vi "Assert Greater_Variant.vi"(4 "Execution time (s)":dbl=-1.0, 6 "error code (1)":i32=1, 7 "Label":string, 8 "error in":errorcluster, 10 "Y":variant, 11 "X":variant) -> (0 "error out":errorcluster, 2 "Properties":refnum<class "Properties.Assert.lvclass">)   [LabVIEW 2021, in "Banana.Caraya.lvlib" / "Platano.CarayaTestSuite.lvclass"]
uses:
  Banana.Caraya/Platano.CarayaTestSuite/Platano.CarayaTestSuite.lvclass
  Banana.Caraya/Platano.CarayaTestSuite/Platano.CarayaTestSuite.lvclass/Platano.CarayaTestSuite.ctl
  <vilib>/addons/_JKI Toolkits/Caraya/classes/Assert/Assert.lvclass
  Platano/Platano.lvclass
  Banana/Banana.lvclass
  Banana.Caraya/Properties.Banana/Properties.Banana.lvclass
  AssertCompareValue/AssertCompareValue.lvclass
  <vilib>/addons/_JKI Toolkits/Caraya/classes/Properties.Assert/Properties.Assert.lvclass
  C:/Program Files (x86)/National Instruments/LabVIEW 2021/vi.lib/addons/_JKI Toolkits/Caraya/classes/Properties/Properties.lvclass
  C:/Program Files (x86)/National Instruments/LabVIEW 2021/vi.lib/addons/_JKI Toolkits/Caraya/classes/Properties.Assert/Properties.Assert.lvclass
  C:/Repositories/LVOS/Bananas/lv-src/Bananas/AssertCompareValue/AssertCompareValue.lvclass
  C:/Repositories/LVOS/Bananas/lv-src/Bananas/BananaPeel/BananaPeel.lvclass
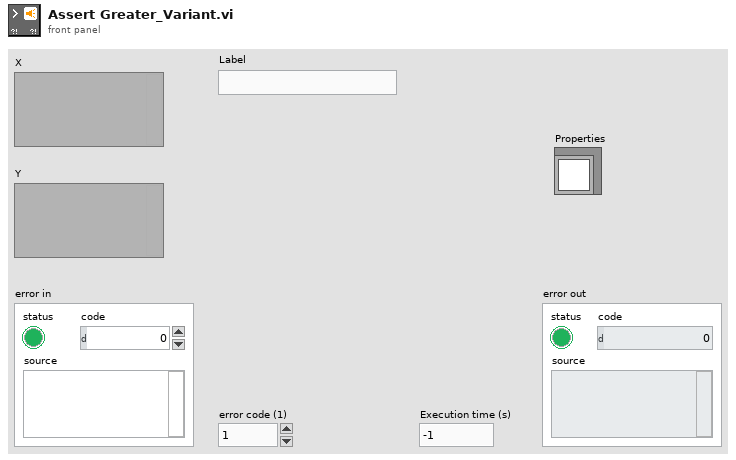
[diagram p1: front panel]
types:
  T1 = typedef "Bananas.lvlib/Assertion Strategies -- cluster.ctl" = cluster{"AssertTrue":refnum<class "AssertTrue.lvclass">, "AssertFalse":refnum<class "AssertFalse.lvclass">, "AssertEqualValue":refnum<class "AssertEqualValue.lvclass">, "AssertEqualType":refnum<class "AssertEqualType.lvclass">, "AssertCompareValue":refnum<class "AssertCompareValue.lvclass">, "AssertError":refnum<class "AssertError.lvclass">, "AssertAlmostEqual":refnum<class "AssertAlmostEqualValue.lvclass">}
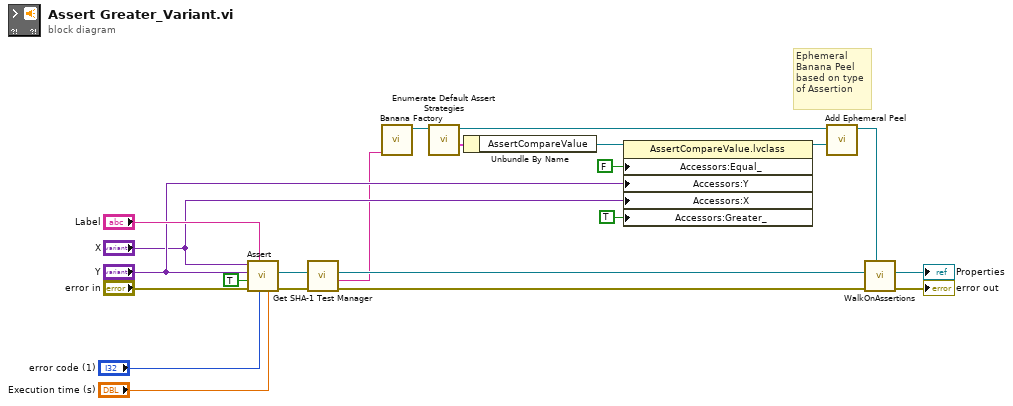
[diagram p0: block diagram]
diagram:
  # "Ephemeral\nBanana Peel\nbased on type\nof Assertion"
  n1 = call-poly <vilib>:"Assert.vi"("Execution time (s)"="Execution time (s)", "error code (1)"="error code (1)", "Label"="Label", "error in (no error)"="error in", "Register with caller test (F)"=TRUE, "Y"="Y", "X"="X") -> ("error out"=w4:errorcluster, "Properties.Assert"=w6:refnum<class "Properties.Assert.lvclass">)  [unwired: 3 in]
  n2 = call "Get SHA-1 Test Manager.vi"("error in (no error)"=w4, "Properties"=w6) -> ("error out"=w3:errorcluster, "SHA-1 hash"=w2:string, "Properties"=w5:refnum<class "Properties.Assert.lvclass">)  [unwired: 7 in]
  n3 = call "Banana Factory.vi"("Varietal"=w2) -> ("Banana"=w1:refnum<class "Banana.lvclass">)  [unwired: 10 in]
  n4 = call "Enumerate Default Assert Strategies.vi"("Banana"=w1) -> ("Strategies"=w9:T1, "Banana"=w14:refnum<class "Banana.lvclass">)  [unwired: 9 in]
  n5 = Unbundle By Name(w9) -> ("AssertCompareValue"=w13:refnum<class "AssertCompareValue.lvclass">)
  n6 = property class="AssertCompareValue.lvclass"(reference=w13, "Accessors:Equal_"=FALSE ("Equal_"), "Accessors:Y"="Y", "Accessors:X"="X", "Accessors:Greater_"=TRUE ("Greater_")) -> (reference out=w10:refnum<class "AssertCompareValue.lvclass">)  [unwired: 1 in, 1 out]
  n7 = call "Add Ephemeral Peel.vi"("BananaPeel"=w10, "Banana"=w14) -> ("Banana"=w15:refnum<class "Banana.lvclass">)  [unwired: 8 in, 1 out]
  n8 = call "WalkOnAssertions.vi"("Banana"=w15, "error in (no error)"=w3, "Properties"=w5) -> ("error out"=→"error out":errorcluster, "Properties out"=→"Properties":refnum<class "Properties.Assert.lvclass">)  [unwired: 7 in]
